vi "ActivateVelocityMode.vi"(4 "error in (no error)":errorcluster, 7 "axis in":cluster{"keyHandle":u32, "nodeId":u16}={"keyHandle"=0, "nodeId"=1}) -> (0 "error out":errorcluster, 3 "axis out":cluster{"keyHandle":u32, "nodeId":u16}={"keyHandle"=0, "nodeId"=1})   [LabVIEW 2010]
doc: "<B>ActivateVelocityMode</B> changes the operational mode to velocity mode (VM)."
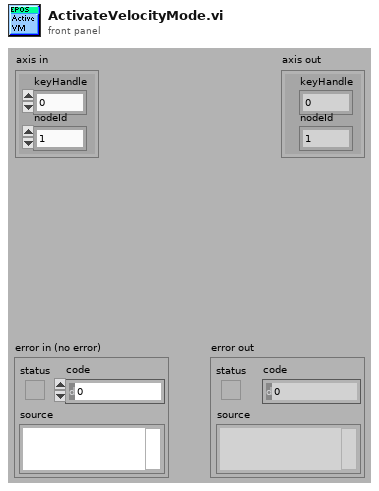
[diagram p1: front panel]
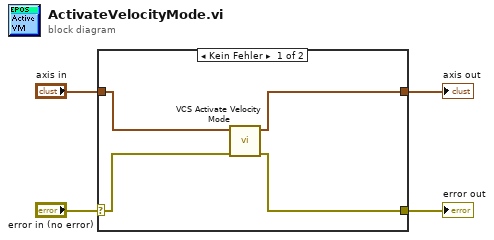
[diagram p0: block diagram]
diagram:
  n1 = case shown="Kein Fehler" "error in (no error)" {
    selector: "error in (no error)" -> [w8 w10]
    tunnel: [w7 w10] -> w3
    tunnel: [w6 w9] -> w2
    tunnel: "axis in" -> [w5 w9]
    frame No Error {
      n2 = call "VCS Activate Velocity Mode.vi"("error in (no error)"=w8, "axis in"=w5) -> ("error out"=w7:errorcluster, "axis out"=w6:cluster{"keyHandle":u32, "nodeId":u16})  [unwired: 8 in]
    }
    frame Error {
    }
  }
  "error out" <- w3
  "axis out" <- w2
